vi "Move Frame.vi"(8 "error in (no error)":errorcluster, 10 "Position":T1, 11 "Test Node View in":refnum<class "Test Node View.lvclass">) -> (0 "error out":errorcluster, 3 "Test Node View out":refnum<class "Test Node View.lvclass">)   [LabVIEW 2013, in "Test Node View.lvlib" / "Test Node View.lvclass"]
uses:
  Test Node View.lvclass
  <vilib>/Utility/miscctls.llb/LVPositionTypeDef.ctl
  Test Node View.lvclass/Test Node View.ctl
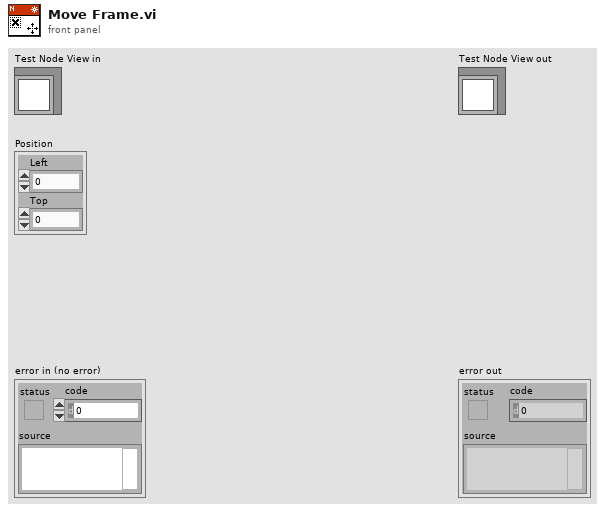
[diagram p1: front panel]
types:
  T1 = typedef "LVPositionTypeDef.ctl" = cluster{"Left":i32, "Top":i32}
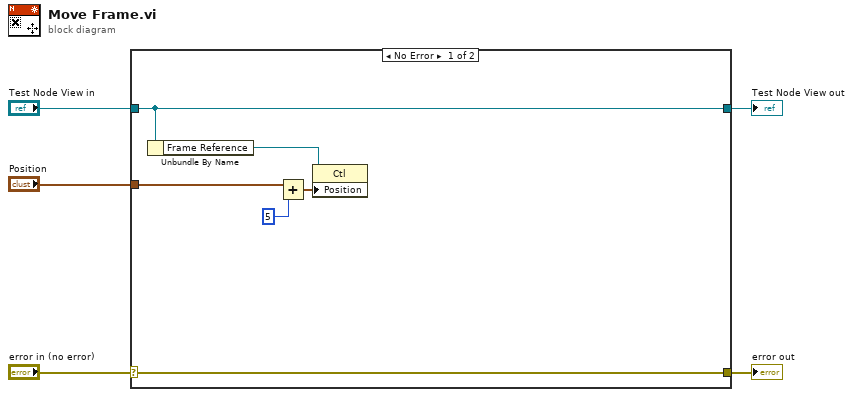
[diagram p0: block diagram]
diagram:
  n1 = case shown="No Error" "error in (no error)" {
    selector: "error in (no error)" -> [w11 w13]
    tunnel: [w11 w13] -> w4
    tunnel: [w10 w12] -> w2
    tunnel: "Test Node View in" -> [w10 w12]
    tunnel: "Position" -> [w7 _]
    frame No Error {
      n2 = Unbundle By Name(w10) -> ("Frame Reference"=w9:refnum<vi>)
      n3 = Add(x=w7, y=5) -> (x+y=w8:T1)
      n4 = property class="Ctl"(reference=w9, "Position"=w8) -> ()  [unwired: 1 in, 2 out]
    }
    frame Error {
    }
  }
  "error out" <- w4
  "Test Node View out" <- w2
